vi "Truck Custom Probe.vi"(1 "truck out":refnum<class "Truck.lvclass">) -> (0 "Boolean":bool)   [LabVIEW 2013, in "Truck.lvclass"]
doc: "A custom probe for the class \"Truck.\" By using this probe, you can view selected data members even if the class is locked."
uses:
  Truck.lvclass
  Truck.lvclass/Truck.ctl
panel:
  out "total cargo capacity":dbl
  out "Bed cargo capacity":dbl format="%#.9f"
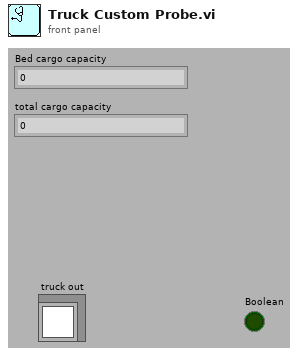
[diagram p1: front panel]
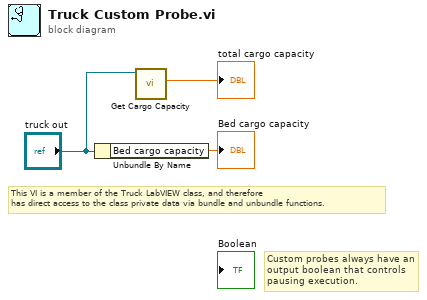
[diagram p0: block diagram]
diagram:
  # "Custom probes always have an\noutput boolean that controls \npausing execution."
  # "This VI is a member of the Truck LabVIEW class, and therefore\nhas direct access to the class private data via bundle and unbundle functions."
  n1 = Unbundle By Name("truck out") -> ("Bed cargo capacity"=→"Bed cargo capacity":dbl)
  n2 = call-dynamic "Get Cargo Capacity.vi"("truck"="truck out") -> ("cargo capacity"=→"total cargo capacity":dbl)  [unwired: 9 in, 1 out]
